vi "calcNewOutputs.vi"(8 "error in (no error)":errorcluster, 10 "outputData":T1 {"Step & Direction" min=-32767}, 11 "FrontPanelValuesSimple in":refnum<class "FrontPanelValuesSimple.lvclass">) -> (0 "error out":errorcluster, 2 "outputData 2":T1 {"Step & Direction" min=-32767}, 3 "FrontPanelValuesSimple out":refnum<class "FrontPanelValuesSimple.lvclass">)   [LabVIEW 2013, in "FrontPanelValuesSimple.lvclass"]
uses:
  FrontPanelValuesSimple.lvclass
  <userlib>/Common/ILC/Typedefs/OutputData.ctl
  <userlib>/Common/ILC/Typedefs/ILCTypedefs.lvlib
panel:
  # "DAC"
  # "DAC"
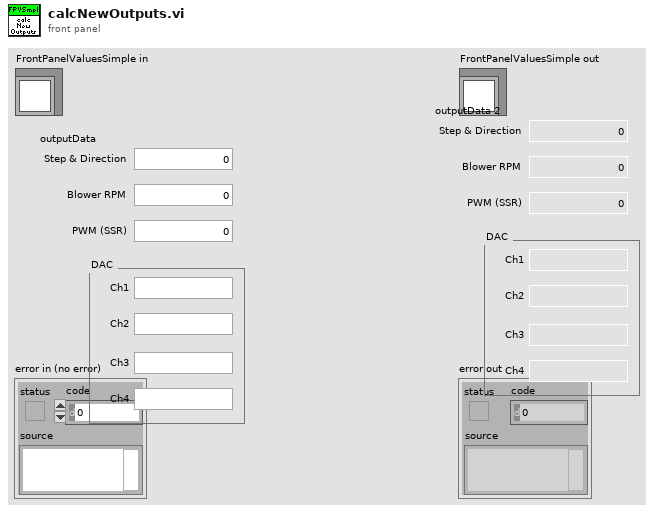
[diagram p1: front panel]
types:
  T1 = typedef "ILCCommon.lvlib/ILCTypedefs.lvlib/OutputData.ctl" = cluster{"Step & Direction":i16, "Blower RPM":u8, "PWM (SSR)":u8, "Ch1":u16, "Ch2":u16, "Ch3":u16, "Ch4":u16}
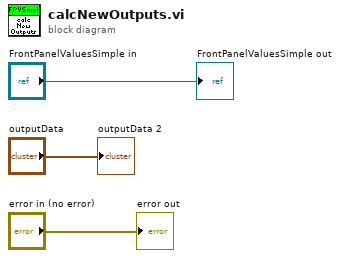
[diagram p0: block diagram]
diagram:
  "error out" <- "error in (no error)"
  "FrontPanelValuesSimple out" <- "FrontPanelValuesSimple in"
  "outputData 2" <- "outputData"
